vi "Left Pre-Buffer Motion Profile Points.vi"(0 "Motor Name":string="Left Drive Master", 5 "Time Conversion Factor":dbl=60.0, 7 "Linear Conversion Factor":dbl=0.32, 9 "Motion Profile Array":dbl[][](array[numeric])=[[0.0, -0.0, 40.0], [0.08329198842021841, 0.0033316795368087365, 40.0], [0.13871006476723616, 0.008880082127498183, 40.0], [0.19396433303999447, 0.016638655449097962, 40.0], [0.24899134067464465, 0.02659830907608375, 40.0], [0.30372956701391185, 0.038747491756640225, 40.0], [0.3581197853422398, 0.05307228317032982, 40.0], [0.41210529675098095, 0.06955649504036905, 40.0], [0.46563202201226506, 0.08818177592085966, 40.0], [0.5186484456210017, 0.10892771374569972, 40.0], [0.5711054118396414, 0.13177193021928538, 40.0], [0.6229557868008607, 0.1566901616913198, 40.0], [0.6741539991903444, 0.18365632165893359, 40.0], [0.7246554880735095, 0.21264254118187398, 40.0], [0.7744160963361527, 0.2436191850353201, 40.0], [0.8233914427397412, 0.27655484274490977, 40.0], [0.871536344702626, 0.31141629653301484, 40.0], [0.9188043401252545, 0.348168470138025, 40.0], [0.9651474165797996, 0.38677436680121696, 40.0], [1.010516036465393, 0.4271950082598327, 40.0], [1.0548596209361827, 0.46938939309728, 40.0], [1.098127647495084, 0.5133144989970834, 40.0], [1.1402716095766003, 0.5589253633801474, 40.0], [1.1812480973316675, 0.6061752872734141, 40.0], [1.2210233487232447, 0.6550162212223438, 40.0], [1.2595796271666686, 0.7053994063090105, 40.0], [1.2969238236836618, 0.7572763592563571, 40.0], [1.3089756274368525, 0.8096353843538312, 40.0], [1.296744128808957, 0.8615051495061895, 40.0], [1.284920488606635, 0.912901969050455, 40.0], [1.2736274263221952, 0.9638470661033428, 40.0], [1.263003625963523, 1.0143672111418838, 40.0], [1.253199706688184, 1.0644951994094112, 40.0], [1.2443727164061194, 1.1142701080656559, 40.0], [1.2366792610760415, 1.1637372785086975, 40.0], [1.2302675826993519, 1.2129479818166715, 40.0], [1.2252691241335159, 1.2619587467820121, 40.0], [1.221790298576604, 1.3108303587250763, 40.0], [1.2199052793414096, 1.3596265698987327, 40.0], [1.2196506062474497, 1.4084125941486307, 40.0], [1.221022244549879, 1.457253483930626, 40.0], [1.2239754539480208, 1.5062125020885468, 40.0], [1.2284274764175083, 1.5553496011452472, 40.0], [1.234262699647989, 1.6047201091311667, 40.0], [1.2413396688338738, 1.6543736958845217, 40.0], [1.249499151502684, 1.7043536619446291, 40.0], [1.2585724332752164, 1.7546965592756378, 40.0], [1.268389109949665, 1.8054321236736244, 40.0], [1.2787838263106184, 1.8565834767260492, 40.0], [1.2896016243434087, 1.9081675416997856, 40.0], [1.300701775709367, 1.9601956127281603, 40.0], [1.3119601492891377, 2.012674018699726, 40.0], [1.3232702871141182, 2.0656048301842906, 40.0], [1.334543425907366, 2.118986567220585, 40.0], [1.3457077282990448, 2.1728148763525468, 40.0], [1.3567069756906882, 2.2270831553801744, 40.0], [1.367498933823948, 2.2817831127331325, 40.0], [1.3778228199704359, 2.3368960255319497, 40.0], [1.362082887563842, 2.3913793410345034, 40.0], [1.3197896354202552, 2.4441709264513136, 40.0], [1.276227779303217, 2.4952200376234424, 40.0], [1.231490219773287, 2.544479646414374, 40.0], [1.1856667253504545, 2.591906315428392, 40.0], [1.1388424028272675, 2.637460011541483, 40.0], [1.0910969572487252, 2.681103889831432, 40.0], [1.042504476426185, 2.7228040688884794, 40.0], [0.9931335515149655, 2.762529410949078, 40.0], [0.9430475978138158, 2.800251314861631, 40.0], [0.8923052835712787, 2.835943526204482, 40.0], [0.8409610070914224, 2.869581966488139, 40.0], [0.7890653803202516, 2.901144581700949, 40.0], [0.7366656940508008, 2.930611209462981, 40.0], [0.6838063521223436, 2.9579634635478746, 40.0], [0.6305292654507303, 2.983184634165904, 40.0], [0.5768742041299887, 3.0062596023311032, 40.0], [0.5228791094609518, 3.027174766709541, 40.0], [0.46858036627928, 3.0459179813607125, 40.0], [0.41401304160254443, 3.0624785030248143, 40.0], [0.3592110929238312, 3.0768469467417674, 40.0], [0.30420755061122323, 3.0890152487662164, 40.0], [0.24903467896883547, 3.09897663592497, 40.0], [0.19372412000617106, 3.1067256007252166, 40.0], [0.13830702342184714, 3.1122578816620905, 40.0], [0.08281416616993595, 3.1155704483088877, 40.0], [0.02752630113267524, 3.1166715003541947, 40.0], [0.0, 3.1166715003541947, 40.0]], 11 "PIDF Profile Slot Select":u8, 12 "Clear Buffer":bool=TRUE) -> (4 "Ready to Execute":bool)   [LabVIEW 2016]
uses:
  <vilib>/Rock Robotics/WPI/ThirdParty/CanMotor/TalonSRX/WPI_CANTalonSRX_APIControlMode.ctl
  <vilib>/Rock Robotics/WPI/ThirdParty/CanMotor/TalonSRX/WPI_CANTalonSRX_GlobalOps.ctl
  <vilib>/Rock Robotics/WPI/ThirdParty/CanMotor/TalonSRX/WPI_CANTalonSRX_MotionProfileTrajectoryPt.ctl
  Global Variables/MotionProfile.vi
panel:
  out "Initialize Loop Index":i32=86
  out "Initialize Is Last":bool=TRUE
  out "Initialize Mot Prof Count":i32=85
  out "Initialize Mot Prof Buffer Is Full":bool
  out "Total Points in File":i32=86
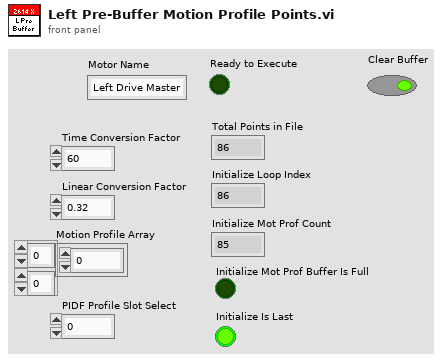
[diagram p1: front panel]
types:
  T1 = typedef "WPI_CANTalonSRX_GlobalOps.ctl" = enum16{"Read For Send", "Write After Receive General", "Write After Receive Feedback", "Write After Receive Encoder", "Write After Receive Ain", "Write Error", "Get All", "Set Output", "Set Mode", "Set Master ID", "Set Brake Mode", "Set Reverse Feedback Sensor", "Set Reverse Closed Loop Output", "Set Override Limits", "Set Forward Limit Enabled", "Set Reverse Limit Enabled", "Set Feedback Select", "Set Profile Select", "Set Throttle Ramp Rate", "Disable", "Set Enc Codes Per Rev", "Set Num Pot Turns", "Set Control Frame Rate", "Enable Legacy Control", "Write After Receive Pulse Width", "Set Enable Frame Rate", "Write After Receive Motion Profile", "Set Motion Profile Flow Control", "Set Motion Profile Control Frame Rate", "Set Current Limit Enable", "Set Usage Frame"}
  T2 = typedef "WPI_CANTalonSRX_APIControlMode.ctl" = enum8{"Percent VBus", "Speed", "Position", "Slave", "Unchanged / Invalid", "Voltage Compensation", "Current", "Motion Profile", "Motion Magic"}
  T3 = typedef "WPI_MotorControlDeviceRef.ctl" = cluster{"DeviceStatus":errorcluster, "Type":T4, "PWM":cluster{"PWM Channel":T5, "DeadBand":T6}, "CAN":cluster{"Device Number":u8, "SetOutput VI Ref":variant, "GetOutput VI Ref":variant, "Enable VI Ref":variant, "Disable VI Ref":variant, "Data":variant}, "Invert":bool}
  T4 = typedef "WPI_MotorControlType.ctl" = enum16{"PWM", "CAN"}
  T5 = typedef "FPGA_DIOPWMChannel.ctl" = enum8{"PWM 0", "PWM 1", "PWM 2", "PWM 3", "PWM 4", "PWM 5", "PWM 6", "PWM 7", "PWM 8", "PWM 9", "PWM MXP 0", "PWM MXP 1", "PWM MXP 2", "PWM MXP 3", "PWM MXP 4", "PWM MXP 5", "PWM MXP 6", "PWM MXP 7", "PWM MXP 8", "PWM MXP 9", "Invalid"}
  T6 = typedef "WPI_PWMDeadband.ctl" = cluster{"Name":string, "maxPositivePwm":i32, "minPositivePwm":i32, "centerPwm":i32, "maxNegativePwm":i32, "minNegativePwm":i32, "angularRange":u16}
  T7 = typedef "WPI_CANTalonSRX_MotionProfileTrajectoryPt.ctl" = cluster{"Duration Ms":u8, "Velocity":dbl, "Position":dbl, "Profile Slot Select":u8, "Is Last":bool, "Velocity Only":bool, "Zero Position":bool, "Compress Code":u8, "Same Velocity":i32, "Delta Position":i32, "Count":u8}
  T8 = typedef "MotionProfile TypeDef.ctl" = cluster{"Left MP Array":dbl[][], "Left MP Index":dbl, "Semaphore":bool, "Right MP Array":dbl[][], "Right MP Index":dbl}
  T9 = typedef "WPI_CANTalonSRX_GlobalStatus.ctl" = cluster{"Applied Throttle":dbl, "Module Enabled":bool, "CAN Error":errorcluster, "Closed Loop Error":dbl, "Forward Limit Switch Closed":bool, "Reverse Limit Switch Closed":bool, "Sensor Position":dbl, "Sensor Velocity":dbl, "Current":dbl, "Sticky Fault - Over Temp":bool, "Sticky Fault - Under Voltage":bool, "Sticky Fault - Forward Limit":bool, "Sticky Fault - Reverse Limit":bool, "Sticky Fault - Forward Soft Limit":bool, "Sticky Fault - Reverse Soft Limit":bool, "Brake is Enabled":bool, "Encoder Position":dbl, "Encoder Velocity":dbl, "Encoder Index Count":dbl, "Encoder A Pin State":bool, "Encoder B Pin State":bool, "Encoder Index Pin State":bool, "Analog In":dbl, "Analog In Velocity":dbl, "Temperature (C)":dbl, "Battery Voltage":dbl, "Control 5 Is Supported":bool, "Current Profile Slot Select":dbl, "Pos Div 8":bool, "Vel Div 4":bool, "Pulse Width Position":i32, "Pulse Width Velocity":i32, "Pulse Width Rise To Rise (us)":i32, "Pulse Width Rise To Fall (us)":i32, "Mot Prof Active Is Under Run":bool, "Mot Prof Active Has Under Run":bool, "Mot Prof Active Is Last":bool, "Mot Prof Active Velocity Only":bool, "Mot Prof Active Is Valid":bool, "Mot Prof Buffer Is Full":bool, "Mot Prof Active Profile Slot Select":i32, "Mot Prof NextID":i32, "Mot Prof Count":i32, "Mot Prof Active Velocity":dbl, "Mot Prof Active Position":dbl, "Mot Prof Output Enable":i32, "UsageFrame":u32}
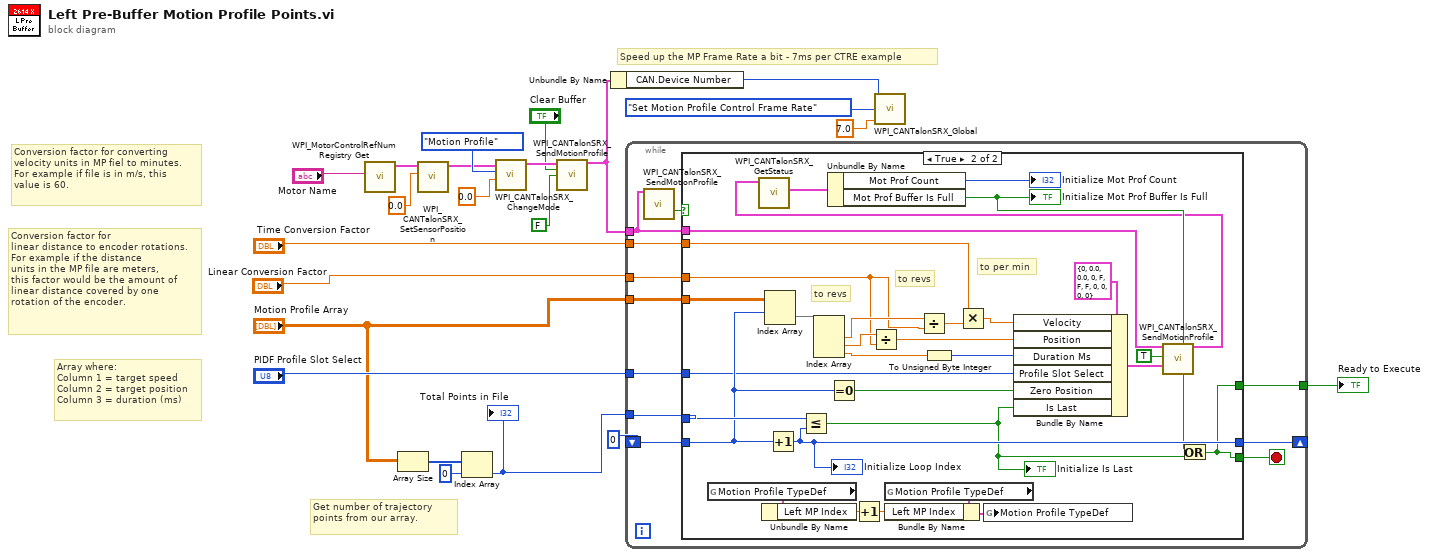
[diagram p0: block diagram]
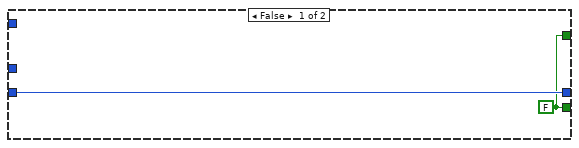
[diagram p2: hidden frame]
diagram:
  # "Array where:\nColumn 1 = target speed\nColumn 2 = target position\nColumn 3 = duration (ms)"
  # "Conversion factor for converting \nvelocity units in MP fiel to minutes.\nFor example if file is in m/s, this\nvalue is 60."
  # "Conversion factor for\nlinear distance to encoder rotations.\nFor example if the distance\nunits in the MP file are meters,\nthis factor would be the amount of\nlinear distance covered by one\nrotation of the encoder."
  # "Speed up the MP Frame Rate a bit - 7ms per CTRE example"
  # "Get number of trajectory points from our array."
  n1 = call <vilib>:"WPI_MotorControlRefNum Registry Get.vi"("refnum name"="Motor Name") -> ("MotorControlDevRef"=w22:T3)  [unwired: 9 in, 1 out]
  n2 = Array Size(array="Motion Profile Array") -> (size(s)=w17:i32[])
  n3 = call <vilib>:"WPI_CANTalonSRX_SetSensorPosition.vi"("New Sensor Position"=0.0, "CAN Talon SRX Ref"=w22) -> ("CAN Talon SRX Ref"=w18:T3)  [unwired: 8 in, 1 out]
  n4 = Index Array(array=w17, index=0) -> (element=w13:i32)
  "Total Points in File" <- w13
  n5 = call <vilib>:"WPI_CANTalonSRX_ChangeMode.vi"("Output"=0.0, "Control Mode"=WPI_CANTalonSRX_APIControlMode."Motion Profile", "CAN Talon SRX Ref"=w18) -> ("CAN Talon SRX Ref"=w15:T3)  [unwired: 7 in, 1 out]
  n6 = call <vilib>:"WPI_CANTalonSRX_SendMotionProfile.vi"("CAN Talon SRX Ref"=w15, "Clear"="Clear Buffer", "Push"=FALSE) -> ("CAN Talon SRX Ref Out"=w11:T3)  [unwired: 9 in, 3 out]
  n7 = Unbundle By Name(w11) -> ("CAN.Device Number"=w10:u8)
  n8 = while {
    tunnel: w11 -> [w26]
    shift-right: [w32] -> _
    shift-left: 0 -> [w30]
    tunnel: w13 -> [w33]
    tunnel: "Motion Profile Array" -> [w31]
    tunnel: "Linear Conversion Factor" -> [w29]
    tunnel: "Time Conversion Factor" -> [w28]
    tunnel: "PIDF Profile Slot Select" -> [w27]
    tunnel: [w23] -> w3
    stop <- w24 stop-if-true
    n9 = call <vilib>:"WPI_CANTalonSRX_SendMotionProfile.vi"("CAN Talon SRX Ref"=w26) -> ("Ready For Next"=w25:bool)  [unwired: 11 in, 3 out]
    n10 = case shown="True" w25 {
      tunnel: w33 -> [_ w66]
      tunnel: [w35 w65] -> w32
      tunnel: w31 -> [_ w59]
      tunnel: w30 -> [w35 w58]
      tunnel: w29 -> [_ w55]
      tunnel: w28 -> [_ w48]
      tunnel: w27 -> [_ w47]
      tunnel: w26 -> [_ w45]
      tunnel: [w34 w43] -> w24
      tunnel: [w34 w43] -> w23
      frame False {
        w34 = FALSE
      }
      frame True {
        # "to per min"
        # "to revs"
        # "to revs"
        n11 = global read "MotionProfile.vi" "Motion Profile TypeDef"() -> (w36:T8)
        n12 = Unbundle By Name(w36) -> ("Left MP Index"=w39:dbl)
        n13 = Index Array(array=w59, index (row)=w58) -> (element=w60:dbl[])  [unwired: 1 in]
        n14 = Increment(x=w58) -> (x+1=w65:i32)
        "Initialize Loop Index" <- w65
        n15 = Less Or Equal?(x=w66, y=w65) -> (x <= y?=w41:bool)
        "Initialize Is Last" <- w41
        n16 = Index Array(array=w60) -> (element #1=w57:dbl, element #2=w56:dbl, element #3=w50:dbl)  [unwired: 3 in]
        n17 = Equal To 0?(x=w58) -> (x = 0?=w62:bool)
        n18 = Increment(x=w39) -> (x+1=w40:dbl)
        n19 = Divide(x=w56, y=w55) -> (x/y=w52:dbl)
        n20 = global read "MotionProfile.vi" "Motion Profile TypeDef"() -> (w37:T8)
        n21 = Bundle By Name(cluster=w37, "Left MP Index"=w40) -> (w38:T8)
        n22 = Divide(x=w57, y=w55) -> (x/y=w54:dbl)
        n23 = To Unsigned Byte Integer(number=w50) -> (unsigned 8bit integer=w49:u8)
        n24 = Multiply(x=w48, y=w54) -> (x*y=w53:dbl)
        n25 = global write "MotionProfile.vi" "Motion Profile TypeDef"(w38) -> ()
        n26 = Bundle By Name(cluster=T7 {"Duration Ms"=0, "Velocity"=0.0, "Position"=0.0, "Profile Slot Select"=0, "Is Last"=FALSE, "Velocity Only"=FALSE, "Zero Position"=FALSE, "Compress Code"=0, "Same Velocity"=0, "Delta Position"=0, "Count"=0} ("New Point"), "Velocity"=w53, "Position"=w52, "Duration Ms"=w49, "Profile Slot Select"=w47, "Zero Position"=w62, "Is Last"=w41) -> (w63:T7)
        n27 = call <vilib>:"WPI_CANTalonSRX_SendMotionProfile.vi"("CAN Talon SRX Ref"=w45, "Push"=TRUE, "New Point"=w63) -> ("CAN Talon SRX Ref Out"=w42:T3)  [unwired: 9 in, 3 out]
        n28 = call <vilib>:"WPI_CANTalonSRX_GetStatus.vi"("CAN Talon SRX Ref"=w42) -> ("Talon SRX Status"=w51:T9)  [unwired: 8 in, 2 out]
        n29 = Unbundle By Name(w51) -> ("Mot Prof Count"=→"Initialize Mot Prof Count":i32, "Mot Prof Buffer Is Full"=w44:bool)
        "Initialize Mot Prof Buffer Is Full" <- w44
        n30 = Or(x=w44, y=w41) -> (x .or. y?=w43:bool)
      }
    }
  }
  "Ready to Execute" <- w3
  n31 = call <vilib>:"WPI_CANTalonSRX_Global.vi"("Set Number"=7.0, "Operation"=WPI_CANTalonSRX_GlobalOps."Set Motion Profile Control Frame Rate", "Device ID (0)"=w10) -> ()  [unwired: 6 in, 3 out]
